vi "Modbus Send Parameters LDO.vi"(8 "error in (no error)":errorcluster, 10 "Array in":i32[](array[numeric]), 11 "Modbus Master in":refnum<class "Modbus Master.lvclass">) -> (0 "error out":errorcluster, 3 "Modbus Master out":refnum<class "Modbus Master.lvclass">)   [LabVIEW 2020, in "Modbus.lvlib"]
uses:
  Modbus.lvlib
  <vilib>/NI/Modbus Library/API/Master/Modbus Master.lvclass
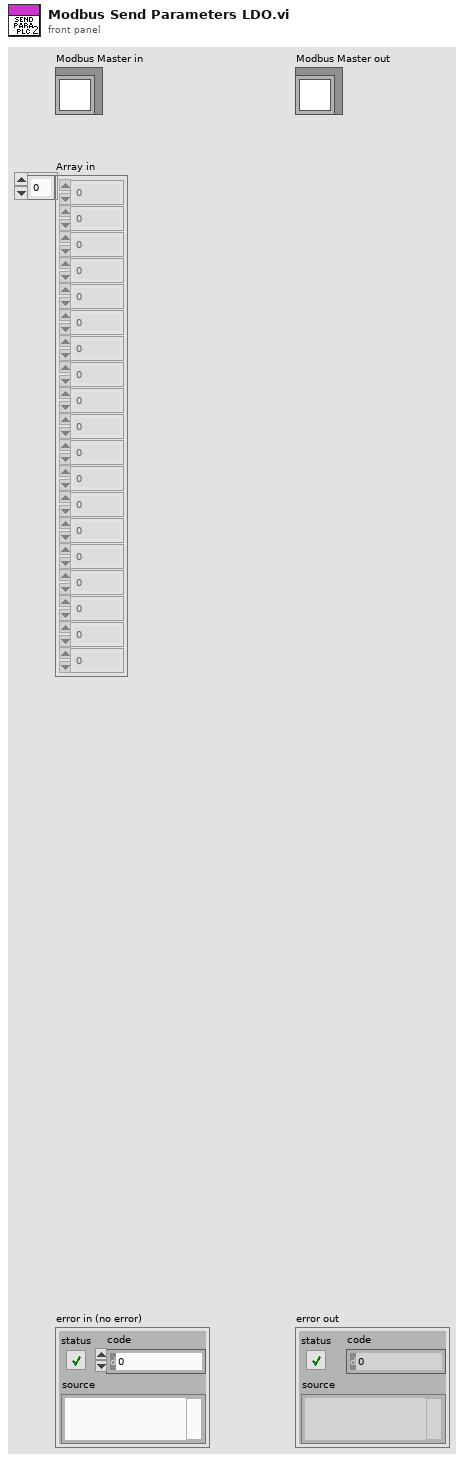
[diagram p1: front panel]
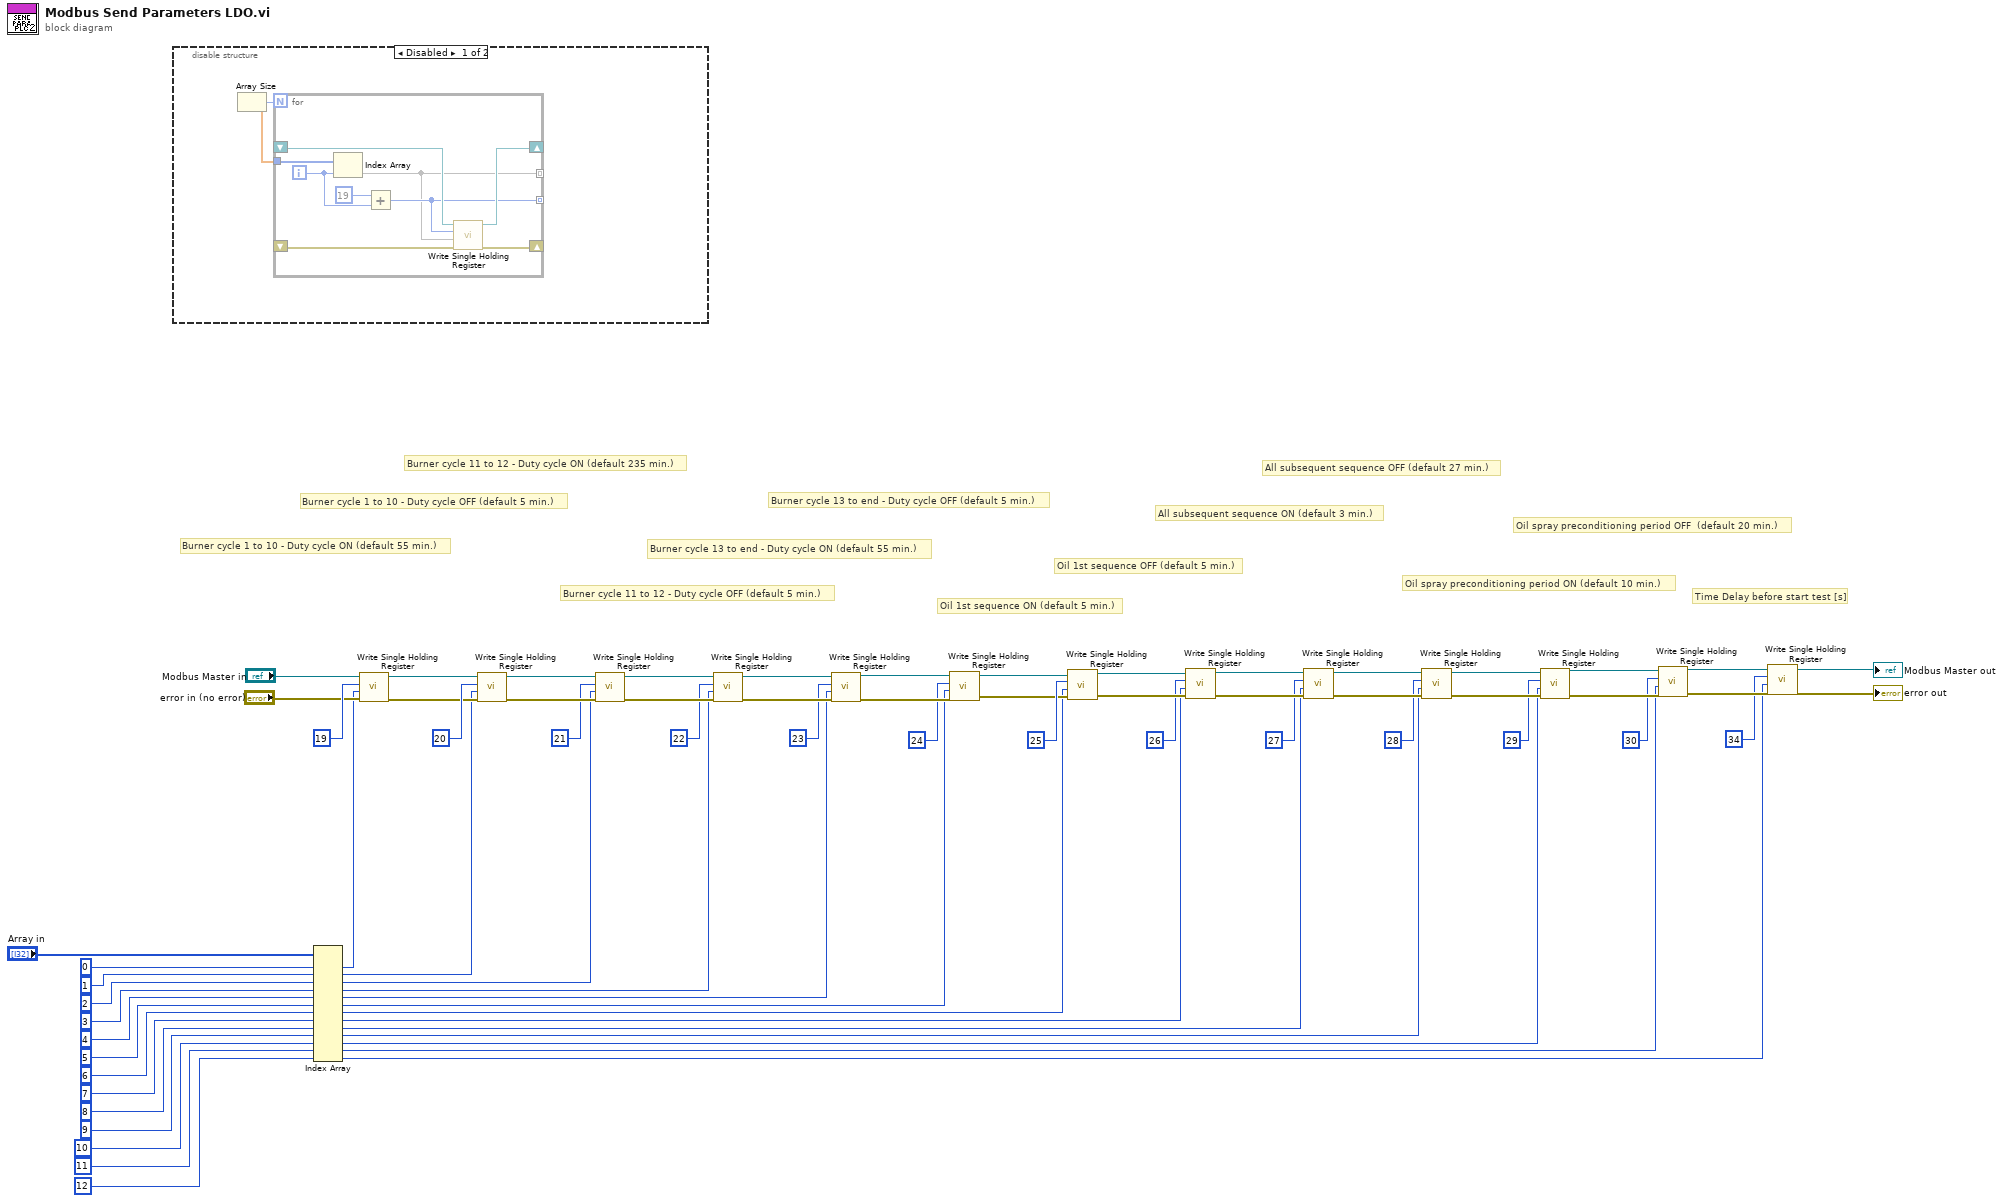
[diagram p0: block diagram]
diagram:
  # "Time Delay before start test [s]"
  # "Oil spray preconditioning period OFF  (default 20 min.)"
  # "Oil spray preconditioning period ON (default 10 min.)"
  # "All subsequent sequence OFF (default 27 min.)"
  # "All subsequent sequence ON (default 3 min.)"
  # "Oil 1st sequence OFF (default 5 min.)"
  # "Oil 1st sequence ON (default 5 min.)"
  # "Burner cycle 13 to end - Duty cycle OFF (default 5 min.)"
  # "Burner cycle 13 to end - Duty cycle ON (default 55 min.)"
  # "Burner cycle 11 to 12 - Duty cycle OFF (default 5 min.)"
  # "Burner cycle 11 to 12 - Duty cycle ON (default 235 min.)"
  # "Burner cycle 1 to 10 - Duty cycle OFF (default 5 min.)"
  # "Burner cycle 1 to 10 - Duty cycle ON (default 55 min.)"
  n1 = disable-structure shown="Disabled" {
    frame Disabled {
      n2 = Array Size() -> (array=w70:dbl[], size(s)=w69:i32)
      n3 = for {
        N: w69 -> [_]
        tunnel: w70 -> [w79]
        shift-right: [w75] -> _
        shift-left: _ -> [w76]
        shift-right: [w73] -> _
        shift-left: _ -> [w74]
        tunnel: [w72] -> _ mode=indexing
        tunnel: [w71] -> _ mode=indexing
        i -> [w78]
        n4 = Index Array(array=w79, index=w78) -> (element=w71)
        n5 = Add(x=19, y=w78) -> (x+y=w72:i32)
        n6 = call-dynamic "Write Single Holding Register.vi"("error in"=w74, "register to write"=w71, "address"=w72, "Modbus master in"=w76) -> ("error out"=w73:errorcluster, "Modbus master out"=w75:refnum<class "Modbus Master.lvclass">)  [unwired: 6 in]
      }
    }
    frame Enabled {
    }
  }
  n7 = Index Array(array="Array in", index #1=0 ("index"), index #2=1 ("index"), index #3=2 ("index"), index #4=3 ("index"), index #5=4 ("index"), index #6=5 ("index"), index #7=6 ("index"), index #8=7 ("index"), index #9=8 ("index"), index #10=9 ("index"), index #11=10 ("index"), index #12=11 ("index"), index #13=12 ("index")) -> (element #1=w13:i32, element #2=w12:i32, element #3=w11:i32, element #4=w10:i32, element #5=w9:i32, element #6=w8:i32, element #7=w7:i32, element #8=w6:i32, element #9=w5:i32, element #10=w4:i32, element #11=w3:i32, element #12=w2:i32, element #13=w1:i32)
  n8 = call-dynamic "Write Single Holding Register.vi"("error in"="error in (no error)", "register to write"=w13, "address"=19 ("x"), "Modbus master in"="Modbus Master in") -> ("error out"=w63:errorcluster, "Modbus master out"=w66:refnum<class "Modbus Master.lvclass">)  [unwired: 6 in]
  n9 = call-dynamic "Write Single Holding Register.vi"("error in"=w63, "register to write"=w12, "address"=20 ("x"), "Modbus master in"=w66) -> ("error out"=w64:errorcluster, "Modbus master out"=w65:refnum<class "Modbus Master.lvclass">)  [unwired: 6 in]
  n10 = call-dynamic "Write Single Holding Register.vi"("error in"=w64, "register to write"=w11, "address"=21 ("x"), "Modbus master in"=w65) -> ("error out"=w61:errorcluster, "Modbus master out"=w59:refnum<class "Modbus Master.lvclass">)  [unwired: 6 in]
  n11 = call-dynamic "Write Single Holding Register.vi"("error in"=w61, "register to write"=w10, "address"=22 ("x"), "Modbus master in"=w59) -> ("error out"=w57:errorcluster, "Modbus master out"=w58:refnum<class "Modbus Master.lvclass">)  [unwired: 6 in]
  n12 = call-dynamic "Write Single Holding Register.vi"("error in"=w57, "register to write"=w9, "address"=23 ("x"), "Modbus master in"=w58) -> ("error out"=w55:errorcluster, "Modbus master out"=w54:refnum<class "Modbus Master.lvclass">)  [unwired: 6 in]
  n13 = call-dynamic "Write Single Holding Register.vi"("error in"=w55, "register to write"=w8, "address"=24 ("x"), "Modbus master in"=w54) -> ("error out"=w47:errorcluster, "Modbus master out"=w52:refnum<class "Modbus Master.lvclass">)  [unwired: 6 in]
  n14 = call-dynamic "Write Single Holding Register.vi"("error in"=w47, "register to write"=w7, "address"=25 ("x"), "Modbus master in"=w52) -> ("error out"=w49:errorcluster, "Modbus master out"=w50:refnum<class "Modbus Master.lvclass">)  [unwired: 6 in]
  n15 = call-dynamic "Write Single Holding Register.vi"("error in"=w49, "register to write"=w6, "address"=26 ("x"), "Modbus master in"=w50) -> ("error out"=w46:errorcluster, "Modbus master out"=w45:refnum<class "Modbus Master.lvclass">)  [unwired: 6 in]
  n16 = call-dynamic "Write Single Holding Register.vi"("error in"=w46, "register to write"=w5, "address"=27 ("x"), "Modbus master in"=w45) -> ("error out"=w42:errorcluster, "Modbus master out"=w43:refnum<class "Modbus Master.lvclass">)  [unwired: 6 in]
  n17 = call-dynamic "Write Single Holding Register.vi"("error in"=w42, "register to write"=w4, "address"=28 ("x"), "Modbus master in"=w43) -> ("error out"=w40:errorcluster, "Modbus master out"=w39:refnum<class "Modbus Master.lvclass">)  [unwired: 6 in]
  n18 = call-dynamic "Write Single Holding Register.vi"("error in"=w40, "register to write"=w3, "address"=29 ("x"), "Modbus master in"=w39) -> ("error out"=w37:errorcluster, "Modbus master out"=w36:refnum<class "Modbus Master.lvclass">)  [unwired: 6 in]
  n19 = call-dynamic "Write Single Holding Register.vi"("error in"=w37, "register to write"=w2, "address"=30 ("x"), "Modbus master in"=w36) -> ("error out"=w19:errorcluster, "Modbus master out"=w18:refnum<class "Modbus Master.lvclass">)  [unwired: 6 in]
  n20 = call-dynamic "Write Single Holding Register.vi"("error in"=w19, "register to write"=w1, "address"=u16 34, "Modbus master in"=w18) -> ("error out"=→"error out":errorcluster, "Modbus master out"=→"Modbus Master out":refnum<class "Modbus Master.lvclass">)  [unwired: 6 in]
